vi "HTML Report Image.vi"(7 "label":string, 9 "image attributes":string, 10 "src - URL of image to embed":string, 11 "HTML in":string) -> (3 "HTML out":string)   [LabVIEW 2015, in "NI_ReportGenerationCore.lvlib"]
doc: "Creates a tag for an embedded image <IMG>.\n\nThe image attributes can be created with \"HTML Image Attribute.vi\"."
uses:
  <vilib>/Utility/NIReport.llb/NI_ReportGenerationCore.lvlib
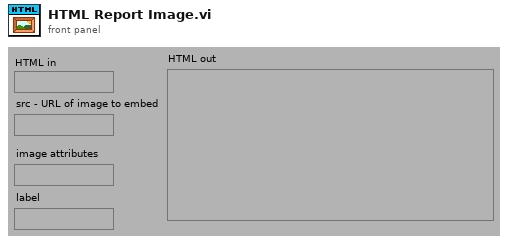
[diagram p1: front panel]
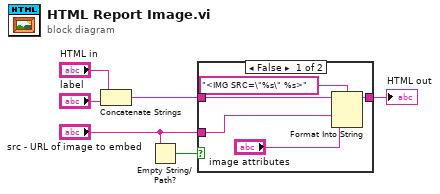
[diagram p0: block diagram]
diagram:
  n1 = Concatenate Strings("HTML in", "label") -> (w1:string)
  n2 = Empty String/Path?(string/path="src - URL of image to embed") -> (empty?=w5:bool)
  n3 = case shown="False" w5 {
    tunnel: "src - URL of image to embed" -> [w8 _]
    tunnel: w1 -> [w10 w12]
    tunnel: [w9 w12] -> w4
    frame False {
      n4 = Format Into String(format string="<IMG SRC=\"%s\" %s>", initial string=w10, w8, "image attributes") -> (resulting string=w9:string)  [unwired: 1 in, 1 out]
    }
    frame True {
    }
  }
  "HTML out" <- w4
